vi "MulticastAnswer (SubVI).vi"(9 "port":u16, 10 "name":string, 11 "data in":string) -> (2 "Array":string[](array[string]), 3 "SUdpAnswer":T1)   [LabVIEW 2017, in "LV_Unicorn.lvlib"]
uses:
  LV_Unicorn.lvlib
  Control/AnswerUDP.ctl
  <vilib>/addons/Tools/Unicode/UTF8 Tools.lvlib
panel:
  out "serverPort":u16
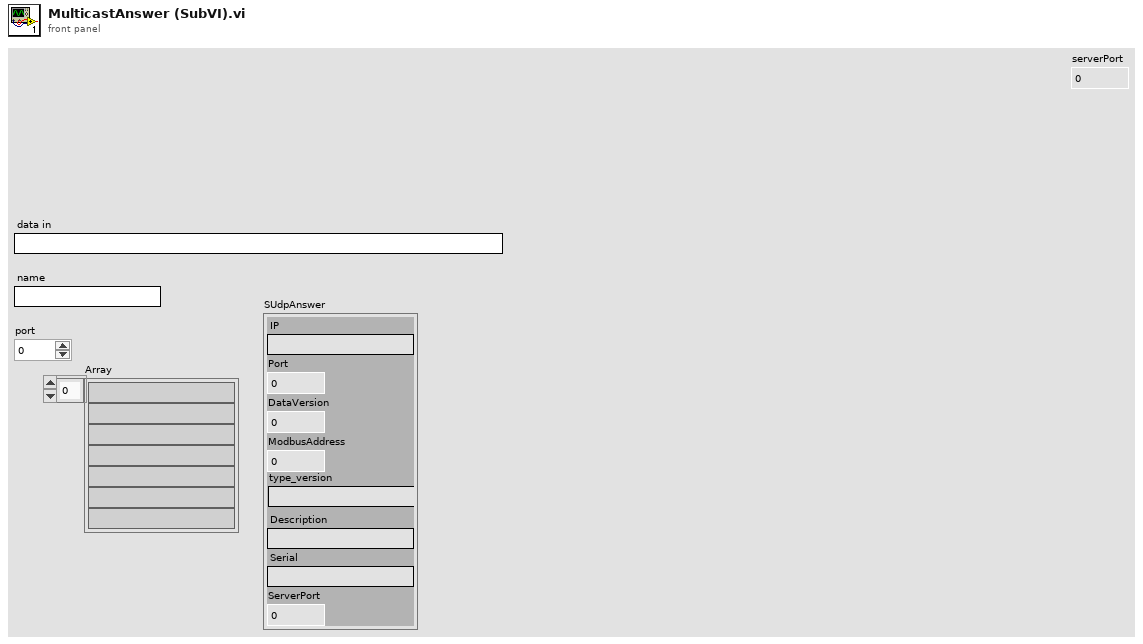
[diagram p1: front panel]
types:
  T1 = typedef "LV_Unicorn.lvlib/AnswerUDP.ctl" = cluster{"IP":string, "Port":u16, "DataVersion":u16, "ModbusAddress":i32, "type_version":string, "Description":string, "Serial":string, "ServerPort":u16}
  T2 = cluster{"magic":u32, "dataVersion":u16, "serverPort":u16, "modbusAddress":i32, "modbustype, version":u32, "description":cluster{"array[0]":u8, "array[1]":u8, "array[2]":u8, "array[3]":u8, "array[4]":u8, "array[5]":u8, "array[6]":u8, "array[7]":u8, "array[8]":u8, "array[0] 2":u8, "array[1] 2":u8, "array[2] 2":u8, "array[3] 2":u8, "array[4] 2":u8, "array[5] 2":u8, "array[6] 2":u8, "array[7] 2":u8, "array[8] 2":u8, "array[0] 3":u8, "array[1] 3":u8, "array[2] 3":u8, "array[3] 3":u8, "array[4] 3":u8, "array[5] 3":u8, "array[6] 3":u8, "array[7] 3":u8, "array[8] 3":u8, "array[0] 4":u8, "array[1] 4":u8, "array[2] 4":u8, "array[3] 4":u8, "array[4] 4":u8, "array[5] 4":u8, "array[6] 4":u8, "array[7] 4":u8, "array[8] 4":u8, "array[0] 5":u8, "array[1] 5":u8, "array[2] 5":u8, "array[3] 5":u8, "array[4] 5":u8, "array[5] 5":u8, "array[6] 5":u8, "array[7] 5":u8, "array[8] 5":u8, "array[0] 6":u8, "array[1] 6":u8, "array[2] 6":u8, "array[3] 6":u8, "array[4] 6":u8, "array[5] 6":u8, "array[6] 6":u8, "array[7] 6":u8, "array[8] 6":u8, "array[0] 7":u8, "array[1] 7":u8, "array[2] 7":u8, "array[3] 7":u8, "array[4] 7":u8, "array[5] 7":u8, "array[6] 7":u8, "array[7] 7":u8, "array[8] 7":u8, "array[0] 8":u8, "array[1] 8":u8, "array[2] 8":u8, "array[3] 8":u8, "array[4] 8":u8, "array[5] 8":u8, "array[6] 8":u8, "array[7] 8":u8, "array[8] 8":u8, "array[0] 9":u8, "array[1] 9":u8, "array[2] 9":u8, "array[3] 9":u8, "array[4] 9":u8, "array[5] 9":u8, "array[6] 9":u8, "array[7] 9":u8, "array[8] 9":u8, "array[0] 10":u8, "array[1] 10":u8, "array[2] 10":u8, "array[3] 10":u8, "array[4] 10":u8, "array[5] 10":u8, "array[6] 10":u8, "array[7] 10":u8, "array[8] 10":u8, "array[0] 11":u8, "array[1] 11":u8, "array[2] 11":u8, "array[3] 11":u8, "array[4] 11":u8, "array[5] 11":u8, "array[6] 11":u8, "array[7] 11":u8, "array[8] 11":u8, "array[8] 12":u8}, "serialNumber":cluster{"array[0]":u8, "array[1]":u8, "array[2]":u8, "array[3]":u8, "array[4]":u8, "array[5]":u8, "array[6]":u8, "array[7]":u8, "array[8]":u8, "array[0] 2":u8, "array[1] 2":u8, "array[2] 2":u8, "array[3] 2":u8, "array[4] 2":u8, "array[5] 2":u8, "array[6] 2":u8, "array[7] 2":u8, "array[8] 2":u8, "array[0] 3":u8, "array[1] 3":u8, "array[2] 3":u8, "array[3] 3":u8, "array[4] 3":u8, "array[5] 3":u8, "array[6] 3":u8, "array[7] 3":u8, "array[8] 3":u8, "array[0] 4":u8, "array[1] 4":u8, "array[2] 4":u8, "array[3] 4":u8, "array[4] 4":u8, "array[5] 4":u8, "array[6] 4":u8, "array[7] 4":u8, "array[8] 4":u8, "array[0] 5":u8, "array[1] 5":u8, "array[2] 5":u8, "array[3] 5":u8}}
  T3 = cluster{"array[0]":u8, "array[1]":u8, "array[2]":u8, "array[3]":u8, "array[4]":u8, "array[5]":u8, "array[6]":u8, "array[7]":u8, "array[8]":u8, "array[0] 2":u8, "array[1] 2":u8, "array[2] 2":u8, "array[3] 2":u8, "array[4] 2":u8, "array[5] 2":u8, "array[6] 2":u8, "array[7] 2":u8, "array[8] 2":u8, "array[0] 3":u8, "array[1] 3":u8, "array[2] 3":u8, "array[3] 3":u8, "array[4] 3":u8, "array[5] 3":u8, "array[6] 3":u8, "array[7] 3":u8, "array[8] 3":u8, "array[0] 4":u8, "array[1] 4":u8, "array[2] 4":u8, "array[3] 4":u8, "array[4] 4":u8, "array[5] 4":u8, "array[6] 4":u8, "array[7] 4":u8, "array[8] 4":u8, "array[0] 5":u8, "array[1] 5":u8, "array[2] 5":u8, "array[3] 5":u8, "array[4] 5":u8, "array[5] 5":u8, "array[6] 5":u8, "array[7] 5":u8, "array[8] 5":u8, "array[0] 6":u8, "array[1] 6":u8, "array[2] 6":u8, "array[3] 6":u8, "array[4] 6":u8, "array[5] 6":u8, "array[6] 6":u8, "array[7] 6":u8, "array[8] 6":u8, "array[0] 7":u8, "array[1] 7":u8, "array[2] 7":u8, "array[3] 7":u8, "array[4] 7":u8, "array[5] 7":u8, "array[6] 7":u8, "array[7] 7":u8, "array[8] 7":u8, "array[0] 8":u8, "array[1] 8":u8, "array[2] 8":u8, "array[3] 8":u8, "array[4] 8":u8, "array[5] 8":u8, "array[6] 8":u8, "array[7] 8":u8, "array[8] 8":u8, "array[0] 9":u8, "array[1] 9":u8, "array[2] 9":u8, "array[3] 9":u8, "array[4] 9":u8, "array[5] 9":u8, "array[6] 9":u8, "array[7] 9":u8, "array[8] 9":u8, "array[0] 10":u8, "array[1] 10":u8, "array[2] 10":u8, "array[3] 10":u8, "array[4] 10":u8, "array[5] 10":u8, "array[6] 10":u8, "array[7] 10":u8, "array[8] 10":u8, "array[0] 11":u8, "array[1] 11":u8, "array[2] 11":u8, "array[3] 11":u8, "array[4] 11":u8, "array[5] 11":u8, "array[6] 11":u8, "array[7] 11":u8, "array[8] 11":u8, "array[8] 12":u8}
  T4 = cluster{"array[0]":u8, "array[1]":u8, "array[2]":u8, "array[3]":u8, "array[4]":u8, "array[5]":u8, "array[6]":u8, "array[7]":u8, "array[8]":u8, "array[0] 2":u8, "array[1] 2":u8, "array[2] 2":u8, "array[3] 2":u8, "array[4] 2":u8, "array[5] 2":u8, "array[6] 2":u8, "array[7] 2":u8, "array[8] 2":u8, "array[0] 3":u8, "array[1] 3":u8, "array[2] 3":u8, "array[3] 3":u8, "array[4] 3":u8, "array[5] 3":u8, "array[6] 3":u8, "array[7] 3":u8, "array[8] 3":u8, "array[0] 4":u8, "array[1] 4":u8, "array[2] 4":u8, "array[3] 4":u8, "array[4] 4":u8, "array[5] 4":u8, "array[6] 4":u8, "array[7] 4":u8, "array[8] 4":u8, "array[0] 5":u8, "array[1] 5":u8, "array[2] 5":u8, "array[3] 5":u8}
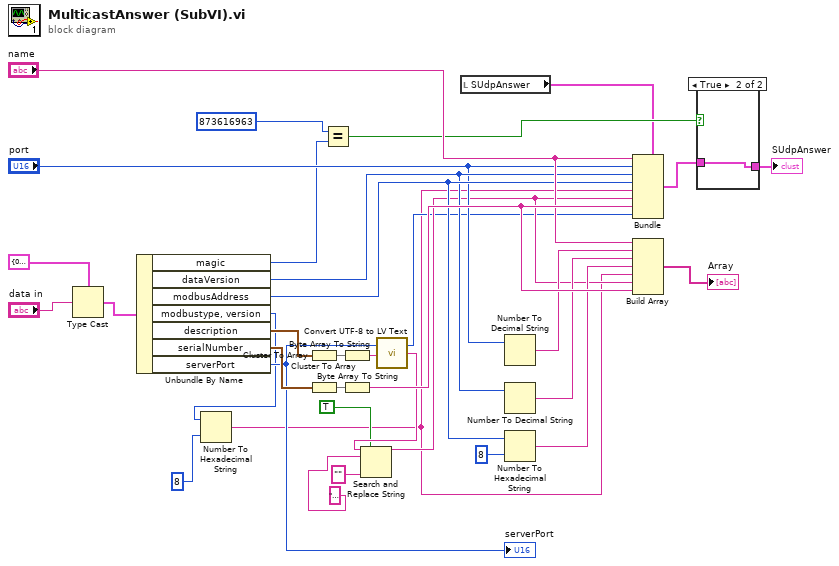
[diagram p0: block diagram]
diagram:
  n1 = Type Cast(type=T2 {"magic"=0, "dataVersion"=0, "serverPort"=0, "modbusAddress"=0, "modbustype, version"=0, "description"={"array[0]"=0, "array[1]"=0, "array[2]"=0, "array[3]"=0, "array[4]"=0, "array[5]"=0, "array[6]"=0, "array[7]"=0, "array[8]"=0, "array[0] 2"=0, "array[1] 2"=0, "array[2] 2"=0, "array[3] 2"=0, "array[4] 2"=0, "array[5] 2"=0, "array[6] 2"=0, "array[7] 2"=0, "array[8] 2"=0, "array[0] 3"=0, "array[1] 3"=0, "array[2] 3"=0, "array[3] 3"=0, "array[4] 3"=0, "array[5] 3"=0, "array[6] 3"=0, "array[7] 3"=0, "array[8] 3"=0, "array[0] 4"=0, "array[1] 4"=0, "array[2] 4"=0, "array[3] 4"=0, "array[4] 4"=0, "array[5] 4"=0, "array[6] 4"=0, "array[7] 4"=0, "array[8] 4"=0, "array[0] 5"=0, "array[1] 5"=0, "array[2] 5"=0, "array[3] 5"=0, "array[4] 5"=0, "array[5] 5"=0, "array[6] 5"=0, "array[7] 5"=0, "array[8] 5"=0, "array[0] 6"=0, "array[1] 6"=0, "array[2] 6"=0, "array[3] 6"=0, "array[4] 6"=0, "array[5] 6"=0, "array[6] 6"=0, "array[7] 6"=0, "array[8] 6"=0, "array[0] 7"=0, "array[1] 7"=0, "array[2] 7"=0, "array[3] 7"=0, "array[4] 7"=0, "array[5] 7"=0, "array[6] 7"=0, "array[7] 7"=0, "array[8] 7"=0, "array[0] 8"=0, "array[1] 8"=0, "array[2] 8"=0, "array[3] 8"=0, "array[4] 8"=0, "array[5] 8"=0, "array[6] 8"=0, "array[7] 8"=0, "array[8] 8"=0, "array[0] 9"=0, "array[1] 9"=0, "array[2] 9"=0, "array[3] 9"=0, "array[4] 9"=0, "array[5] 9"=0, "array[6] 9"=0, "array[7] 9"=0, "array[8] 9"=0, "array[0] 10"=0, "array[1] 10"=0, "array[2] 10"=0, "array[3] 10"=0, "array[4] 10"=0, "array[5] 10"=0, "array[6] 10"=0, "array[7] 10"=0, "array[8] 10"=0, "array[0] 11"=0, "array[1] 11"=0, "array[2] 11"=0, "array[3] 11"=0, "array[4] 11"=0, "array[5] 11"=0, "array[6] 11"=0, "array[7] 11"=0, "array[8] 11"=0, "array[8] 12"=0}, "serialNumber"={"array[0]"=0, "array[1]"=0, "array[2]"=0, "array[3]"=0, "array[4]"=0, "array[5]"=0, "array[6]"=0, "array[7]"=0, "array[8]"=0, "array[0] 2"=0, "array[1] 2"=0, "array[2] 2"=0, "array[3] 2"=0, "array[4] 2"=0, "array[5] 2"=0, "array[6] 2"=0, "array[7] 2"=0, "array[8] 2"=0, "array[0] 3"=0, "array[1] 3"=0, "array[2] 3"=0, "array[3] 3"=0, "array[4] 3"=0, "array[5] 3"=0, "array[6] 3"=0, "array[7] 3"=0, "array[8] 3"=0, "array[0] 4"=0, "array[1] 4"=0, "array[2] 4"=0, "array[3] 4"=0, "array[4] 4"=0, "array[5] 4"=0, "array[6] 4"=0, "array[7] 4"=0, "array[8] 4"=0, "array[0] 5"=0, "array[1] 5"=0, "array[2] 5"=0, "array[3] 5"=0}} ("Cluster 2"), x="data in") -> (*(type *) &x=w14:T2)
  n2 = Unbundle By Name(w14) -> ("magic"=w21:u32, "dataVersion"=w26:u16, "modbusAddress"=w27:i32, "modbustype, version"=w2:u32, "description"=w15:T3, "serialNumber"=w18:T4, "serverPort"=w4:u16)
  "serverPort" <- w4
  n3 = Number To Hexadecimal String(1:i16 8 ("width (-)"), 2:w2) -> (0:w1:string)
  n4 = Cluster To Array(cluster=w15) -> (array=w16:u8[])
  n5 = Cluster To Array(cluster=w18) -> (array=w17:u8[])
  n6 = Equal?(x=u32 873616963 ("magic"), y=w21) -> (x = y?=w24:bool)
  n7 = Byte Array To String(unsigned byte array=w16) -> (string=w19:string)
  n8 = Byte Array To String(unsigned byte array=w17) -> (string=w32:string)
  n9 = call <vilib>:"Convert UTF-8 to LV Text.vi"("UTF-8 Text"=w19) -> ("LV Text"=w10:string)  [unwired: 13 in, 1 out]
  n10 = Search and Replace String(replace all?=TRUE ("replace all? (F)"), input string=w10, search string="\u0000", replace string="" ("replace string (\"\")")) -> (result string=w7:string)  [unwired: 4 in, 3 out]
  n11 = local read "SUdpAnswer"() -> (w5:T1)
  n12 = Number To Decimal String(number="port") -> (decimal integer string=w29:string)  [unwired: 1 in]
  n13 = Number To Decimal String(number=w26) -> (decimal integer string=w30:string)  [unwired: 1 in]
  n14 = Number To Hexadecimal String(1:i16 8 ("width (-)"), 2:w27) -> (0:w31:string)
  n15 = Bundle(cluster=w5, "IP"="name", "Port"="port", "DataVersion"=w26, "ModbusAddress"=w27, "type_version"=w1, "Description"=w7, "Serial"=w32, "ServerPort"=w4) -> (w23:T1)
  n16 = Build Array("name", w29, w30, w31, w1, w7, w32) -> (→"Array":string[])
  n17 = case shown="True" w24 {
    tunnel: [_ w34] -> w22
    tunnel: w23 -> [_ w34]
    frame False {
    }
    frame True {
    }
  }
  "SUdpAnswer" <- w22
